vi "ep_Get EN50160 Limits.vi"(0 "nominal frequency":enum16{"50 Hz", "60 Hz"}(ring), 5 "nominal voltage [V]":dbl=230.0, 7 "signaling frequency [Hz]":dbl=216.66) -> (4 "EN50160 limits":T1={"frequency limits 1"={"upper limit"=50.5, "lower limit"=49.5, "required percentage"=99.5}, "frequency limits 2"={"upper limit"=52.0, "lower limit"=47.0, "required percentage"=100.0}, "voltage magnitude limits 1"={"upper limit"=252.99999999999997, "lower limit"=206.99999999999997, "required percentage"=95.0}, "voltage magnitude limits 2"={"upper limit"=252.99999999999997, "lower limit"=195.49999999999997, "required percentage"=100.0}, "flicker Plt limits"={"upper limit"=1.0, "lower limit"=-inf, "required percentage"=95.0}, "signalling voltage limits"={"upper limit"=20.7, "lower limit"=-inf, "required percentage"=99.0}, "voltage unbalance limits"={"upper limit"=2.0, "lower limit"=0.0, "required percentage"=95.0}, "voltage THD limits"={"upper limit"=8.0, "lower limit"=-inf, "required percentage"=95.0}, "harmonics voltage limits (1..25 harm.)"=[{"upper limit"=inf, "lower limit"=-inf, "required percentage"=95.0}, {"upper limit"=4.6, "lower limit"=-inf, "required percentage"=95.0}, {"upper limit"=11.5, "lower limit"=-inf, "required percentage"=95.0}, {"upper limit"=2.3, "lower limit"=-inf, "required percentage"=95.0}, {"upper limit"=13.799999999999999, "lower limit"=-inf, "required percentage"=95.0}, {"upper limit"=1.15, "lower limit"=-inf, "required percentage"=95.0}, {"upper limit"=11.5, "lower limit"=-inf, "required percentage"=95.0}, {"upper limit"=1.15, "lower limit"=-inf, "required percentage"=95.0}, {"upper limit"=3.4499999999999997, "lower limit"=-inf, "required percentage"=95.0}, {"upper limit"=1.15, "lower limit"=-inf, "required percentage"=95.0}, {"upper limit"=8.049999999999999, "lower limit"=-inf, "required percentage"=95.0}, {"upper limit"=1.15, "lower limit"=-inf, "required percentage"=95.0}, {"upper limit"=6.8999999999999995, "lower limit"=-inf, "required percentage"=95.0}, {"upper limit"=1.15, "lower limit"=-inf, "required percentage"=95.0}, {"upper limit"=1.15, "lower limit"=-inf, "required percentage"=95.0}, {"upper limit"=1.15, "lower limit"=-inf, "required percentage"=95.0}, {"upper limit"=4.6, "lower limit"=-inf, "required percentage"=95.0}, {"upper limit"=1.15, "lower limit"=-inf, "required percentage"=95.0}, {"upper limit"=3.4499999999999997, "lower limit"=-inf, "required percentage"=95.0}, {"upper limit"=1.15, "lower limit"=-inf, "required percentage"=95.0}, {"upper limit"=1.15, "lower limit"=-inf, "required percentage"=95.0}, {"upper limit"=1.15, "lower limit"=-inf, "required percentage"=95.0}, {"upper limit"=3.4499999999999997, "lower limit"=-inf, "required percentage"=95.0}, {"upper limit"=1.15, "lower limit"=-inf, "required percentage"=95.0}, {"upper limit"=3.4499999999999997, "lower limit"=-inf, "required percentage"=95.0}]})   [LabVIEW 2011, in "NI_EP_Power Quality.lvlib"]
uses:
  <vilib>/addons/Electrical Power/PQ/NI_EP_Power Quality.lvlib
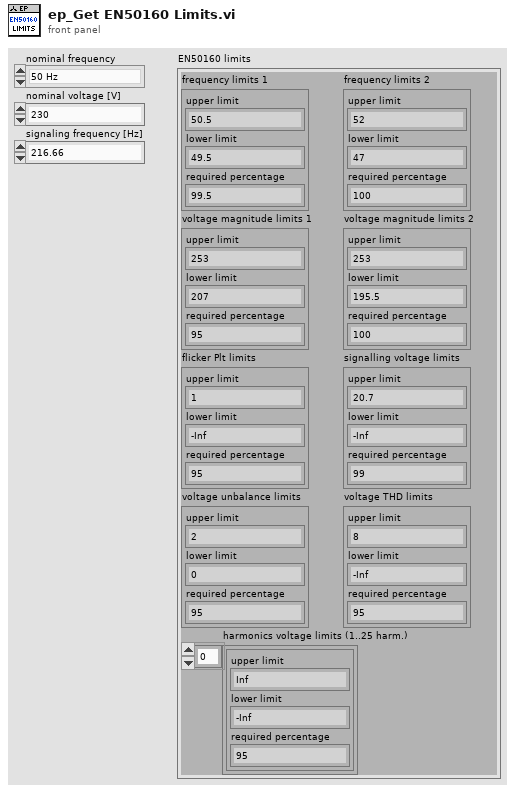
[diagram p1: front panel]
types:
  T1 = cluster{"frequency limits 1":cluster{"upper limit":dbl, "lower limit":dbl, "required percentage":dbl}, "frequency limits 2":cluster{"upper limit":dbl, "lower limit":dbl, "required percentage":dbl}, "voltage magnitude limits 1":cluster{"upper limit":dbl, "lower limit":dbl, "required percentage":dbl}, "voltage magnitude limits 2":cluster{"upper limit":dbl, "lower limit":dbl, "required percentage":dbl}, "flicker Plt limits":cluster{"upper limit":dbl, "lower limit":dbl, "required percentage":dbl}, "signalling voltage limits":cluster{"upper limit":dbl, "lower limit":dbl, "required percentage":dbl}, "voltage unbalance limits":cluster{"upper limit":dbl, "lower limit":dbl, "required percentage":dbl}, "voltage THD limits":cluster{"upper limit":dbl, "lower limit":dbl, "required percentage":dbl}, "harmonics voltage limits (1..25 harm.)":cluster{"upper limit":dbl, "lower limit":dbl, "required percentage":dbl}[]}
  T2 = cluster{"upper limit":dbl, "lower limit":dbl, "required percentage to be in limits":dbl}
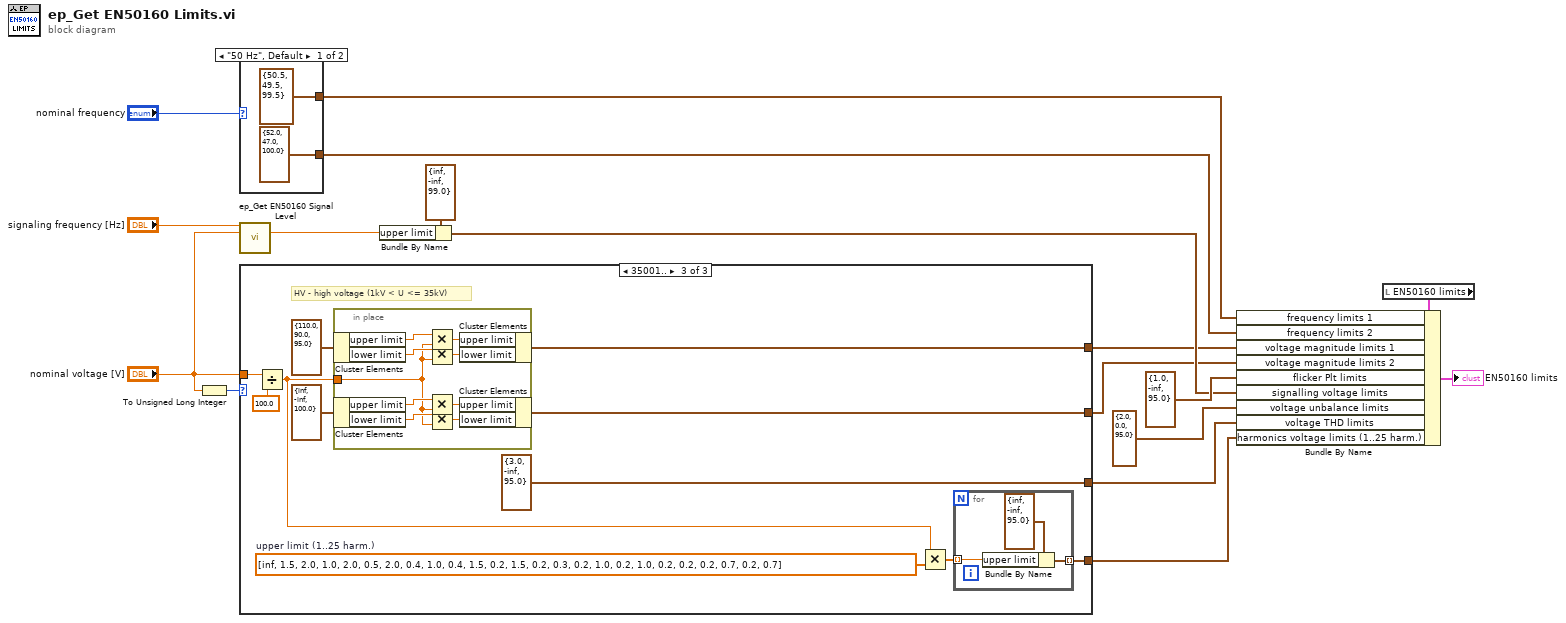
[diagram p0: block diagram]
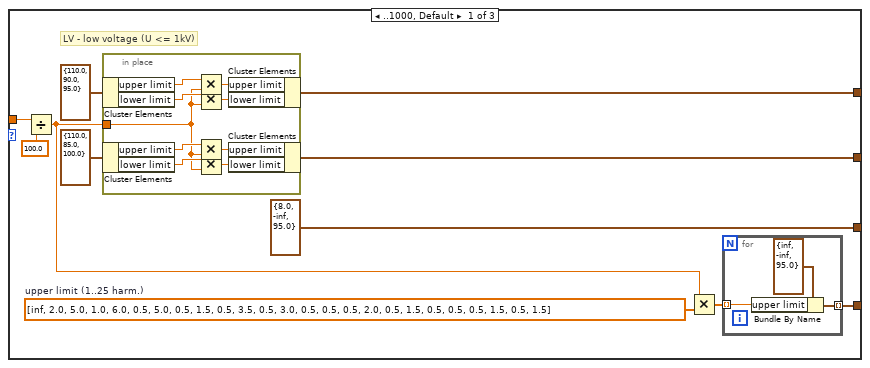
[diagram p2: hidden frame]
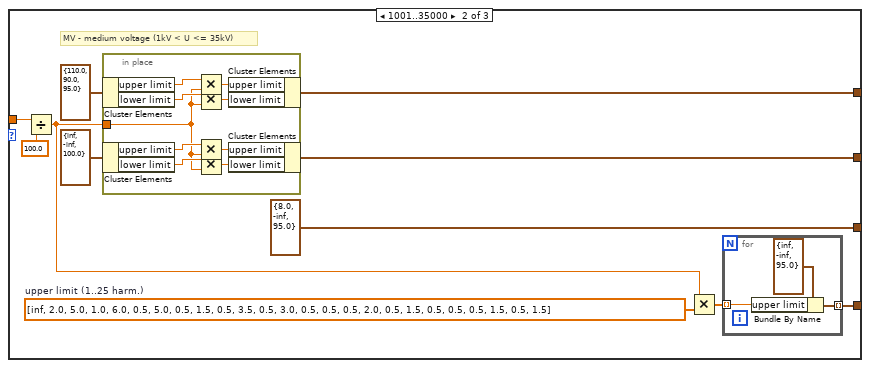
[diagram p3: hidden frame]
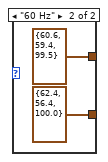
[diagram p4: hidden frame]
diagram:
  n1 = To Unsigned Long Integer(number="nominal voltage [V]") -> (unsigned 32bit integer=w13:u32)
  n2 = case shown="\"50 Hz\", Default" "nominal frequency" {
    tunnel: [T2 {"upper limit"=50.5, "lower limit"=49.5, "required percentage to be in limits"=99.5} ("EN50160 limits") T2 {"upper limit"=60.6, "lower limit"=59.4, "required percentage to be in limits"=99.5} ("EN50160 limits")] -> w10
    tunnel: [T2 {"upper limit"=52.0, "lower limit"=47.0, "required percentage to be in limits"=100.0} ("EN50160 limits") T2 {"upper limit"=62.4, "lower limit"=56.4, "required percentage to be in limits"=100.0} ("EN50160 limits")] -> w9
    frame "50 Hz", Default {
    }
    frame "60 Hz" {
    }
  }
  n3 = call <vilib>:"ep_Get EN50160 Signal Level.vi"("signaling frequency [Hz]"="signaling frequency [Hz]", "nominal voltage [V]"="nominal voltage [V]") -> ("signal level [V]"=w11:dbl)  [unwired: 12 in, 1 out]
  n4 = case shown="35001.." w13 {
    tunnel: "nominal voltage [V]" -> [w29 w52 w75]
    tunnel: [w28 w51 w74] -> w3
    tunnel: [w27 w50 w73] -> w4
    tunnel: [T2 {"upper limit"=8.0, "lower limit"=-inf, "required percentage to be in limits"=95.0} ("EN50160 limits") T2 {"upper limit"=8.0, "lower limit"=-inf, "required percentage to be in limits"=95.0} ("EN50160 limits") T2 {"upper limit"=3.0, "lower limit"=-inf, "required percentage to be in limits"=95.0} ("EN50160 limits")] -> w5
    tunnel: [w23 w46 w70] -> w2
    frame ..1000, Default {
      w24 = dbl[] [inf, 2.0, 5.0, 1.0, 6.0, 0.5, 5.0, 0.5, 1.5, 0.5, 3.5, 0.5, 3.0, 0.5, 0.5, 0.5, 2.0, 0.5, 1.5, 0.5, 0.5, 0.5, 1.5, 0.5, 1.5]  # upper limit (1..25 harm.)
      # "LV - low voltage (U <= 1kV)"
      n5 = Divide(x=w29, y=100.0) -> (x/y=w22:dbl)
      n6 = in-place {
        in-place-border: w22 -> [w40]
        n7 = in-place-cluster #1(T2 {"upper limit"=110.0, "lower limit"=90.0, "required percentage to be in limits"=95.0} ("EN50160 limits")) -> ("upper limit"=w44:dbl, "lower limit"=w43:dbl)
        n8 = in-place-cluster #2(T2 {"upper limit"=110.0, "lower limit"=85.0, "required percentage to be in limits"=100.0} ("EN50160 limits")) -> ("upper limit"=w42:dbl, "lower limit"=w41:dbl)
        n9 = Multiply(x=w44, y=w40) -> (x*y=w39:dbl)
        n10 = Multiply(x=w43, y=w40) -> (x*y=w38:dbl)
        n11 = Multiply(x=w42, y=w40) -> (x*y=w37:dbl)
        n12 = Multiply(x=w41, y=w40) -> (x*y=w36:dbl)
        n13 = in-place-cluster #1("upper limit"=w39, "lower limit"=w38) -> (w27:T2)
        n14 = in-place-cluster #2("upper limit"=w37, "lower limit"=w36) -> (w28:T2)
      }
      n15 = Multiply(x=w22, y=w24) -> (x*y=w25:dbl[])
      n16 = for {
        tunnel: [w34] -> w23 mode=indexing
        tunnel: w25 -> [w33] mode=indexing
        n17 = Bundle By Name(cluster=T2 {"upper limit"=inf, "lower limit"=-inf, "required percentage to be in limits"=95.0} ("EN50160 limits"), "upper limit"=w33) -> (w34:T2)
      }
    }
    frame 1001..35000 {
      w45 = dbl[] [inf, 2.0, 5.0, 1.0, 6.0, 0.5, 5.0, 0.5, 1.5, 0.5, 3.5, 0.5, 3.0, 0.5, 0.5, 0.5, 2.0, 0.5, 1.5, 0.5, 0.5, 0.5, 1.5, 0.5, 1.5]  # upper limit (1..25 harm.)
      # "MV - medium voltage (1kV < U <= 35kV)"
      n18 = Divide(x=w52, y=100.0) -> (x/y=w47:dbl)
      n19 = in-place {
        in-place-border: w47 -> [w63]
        n20 = in-place-cluster #3(T2 {"upper limit"=110.0, "lower limit"=90.0, "required percentage to be in limits"=95.0} ("EN50160 limits")) -> ("upper limit"=w67:dbl, "lower limit"=w66:dbl)
        n21 = in-place-cluster #4(T2 {"upper limit"=inf, "lower limit"=-inf, "required percentage to be in limits"=100.0} ("EN50160 limits")) -> ("upper limit"=w65:dbl, "lower limit"=w64:dbl)
        n22 = Multiply(x=w67, y=w63) -> (x*y=w62:dbl)
        n23 = Multiply(x=w66, y=w63) -> (x*y=w61:dbl)
        n24 = Multiply(x=w65, y=w63) -> (x*y=w60:dbl)
        n25 = Multiply(x=w64, y=w63) -> (x*y=w59:dbl)
        n26 = in-place-cluster #3("upper limit"=w62, "lower limit"=w61) -> (w50:T2)
        n27 = in-place-cluster #4("upper limit"=w60, "lower limit"=w59) -> (w51:T2)
      }
      n28 = Multiply(x=w47, y=w45) -> (x*y=w48:dbl[])
      n29 = for {
        tunnel: [w57] -> w46 mode=indexing
        tunnel: w48 -> [w56] mode=indexing
        n30 = Bundle By Name(cluster=T2 {"upper limit"=inf, "lower limit"=-inf, "required percentage to be in limits"=95.0} ("EN50160 limits"), "upper limit"=w56) -> (w57:T2)
      }
    }
    frame 35001.. {
      w68 = dbl[] [inf, 1.5, 2.0, 1.0, 2.0, 0.5, 2.0, 0.4, 1.0, 0.4, 1.5, 0.2, 1.5, 0.2, 0.3, 0.2, 1.0, 0.2, 1.0, 0.2, 0.2, 0.2, 0.7, 0.2, 0.7]  # upper limit (1..25 harm.)
      # "HV - high voltage (1kV < U <= 35kV)"
      n31 = Divide(x=w75, y=100.0) -> (x/y=w69:dbl)
      n32 = in-place {
        in-place-border: w69 -> [w86]
        n33 = in-place-cluster #5(T2 {"upper limit"=110.0, "lower limit"=90.0, "required percentage to be in limits"=95.0} ("EN50160 limits")) -> ("upper limit"=w90:dbl, "lower limit"=w89:dbl)
        n34 = in-place-cluster #6(T2 {"upper limit"=inf, "lower limit"=-inf, "required percentage to be in limits"=100.0} ("EN50160 limits")) -> ("upper limit"=w88:dbl, "lower limit"=w87:dbl)
        n35 = Multiply(x=w90, y=w86) -> (x*y=w85:dbl)
        n36 = Multiply(x=w89, y=w86) -> (x*y=w84:dbl)
        n37 = Multiply(x=w88, y=w86) -> (x*y=w83:dbl)
        n38 = Multiply(x=w87, y=w86) -> (x*y=w82:dbl)
        n39 = in-place-cluster #5("upper limit"=w85, "lower limit"=w84) -> (w73:T2)
        n40 = in-place-cluster #6("upper limit"=w83, "lower limit"=w82) -> (w74:T2)
      }
      n41 = Multiply(x=w69, y=w68) -> (x*y=w71:dbl[])
      n42 = for {
        tunnel: [w80] -> w70 mode=indexing
        tunnel: w71 -> [w79] mode=indexing
        n43 = Bundle By Name(cluster=T2 {"upper limit"=inf, "lower limit"=-inf, "required percentage to be in limits"=95.0} ("EN50160 limits"), "upper limit"=w79) -> (w80:T2)
      }
    }
  }
  n44 = Bundle By Name(cluster=T2 {"upper limit"=inf, "lower limit"=-inf, "required percentage to be in limits"=99.0} ("EN50160 limits"), "upper limit"=w11) -> (w6:T2)
  n45 = local read "EN50160 limits"() -> (w1:T1)
  n46 = Bundle By Name(cluster=w1, "frequency limits 1"=w10, "frequency limits 2"=w9, "voltage magnitude limits 1"=w4, "voltage magnitude limits 2"=w3, "flicker Plt limits"=T2 {"upper limit"=1.0, "lower limit"=-inf, "required percentage to be in limits"=95.0} ("EN50160 limits"), "signalling voltage limits"=w6, "voltage unbalance limits"=T2 {"upper limit"=2.0, "lower limit"=0.0, "required percentage to be in limits"=95.0} ("EN50160 limits"), "voltage THD limits"=w5, "harmonics voltage limits (1..25 harm.)"=w2) -> (→"EN50160 limits":T1)
